vi "setUp.vi"(8 "error in (no error)":errorcluster, 11 "reference in":refnum<class "DFA Tester.lvclass">) -> (0 "error out":errorcluster, 3 "reference out":refnum<class "DFA Tester.lvclass">)   [LabVIEW 2017, in "DFA Tester.lvclass"]
doc: "setUp runs prior to the test method during test execution. Use this method to initialize any object data required by your tests."
uses:
  DFA Tester.lvclass
  C:/Program Files (x86)/National Instruments/LabVIEW 2017/vi.lib/addons/_JKI Toolkits/VI Tester/TestCase.llb/TestCase.lvclass
  Core/Assert API Components/Failure Actions.ctl
  DFA Tester.lvclass/DFA Tester.ctl
  <vilib>/addons/_JKI Toolkits/VI Tester/TestCase.llb/TestCase.lvclass
  Core/Assert API Components/Assert API Components.lvlib
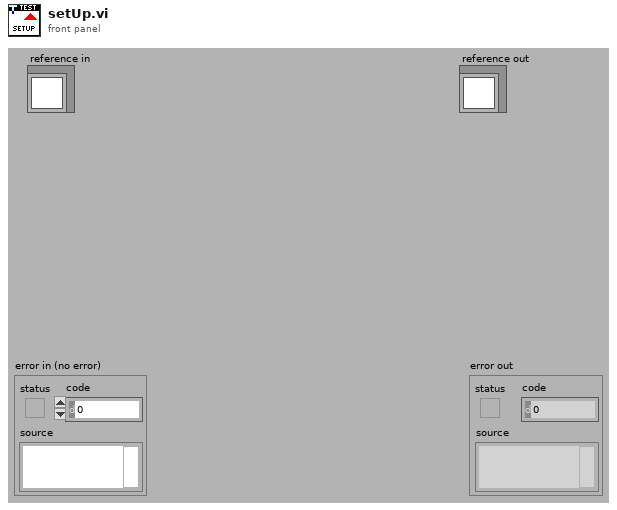
[diagram p1: front panel]
types:
  T1 = typedef "Assert API Components.lvlib/Failure Actions.ctl" = enum16{"None", "Log To File", "Pause Execution", "Abort Execution"}
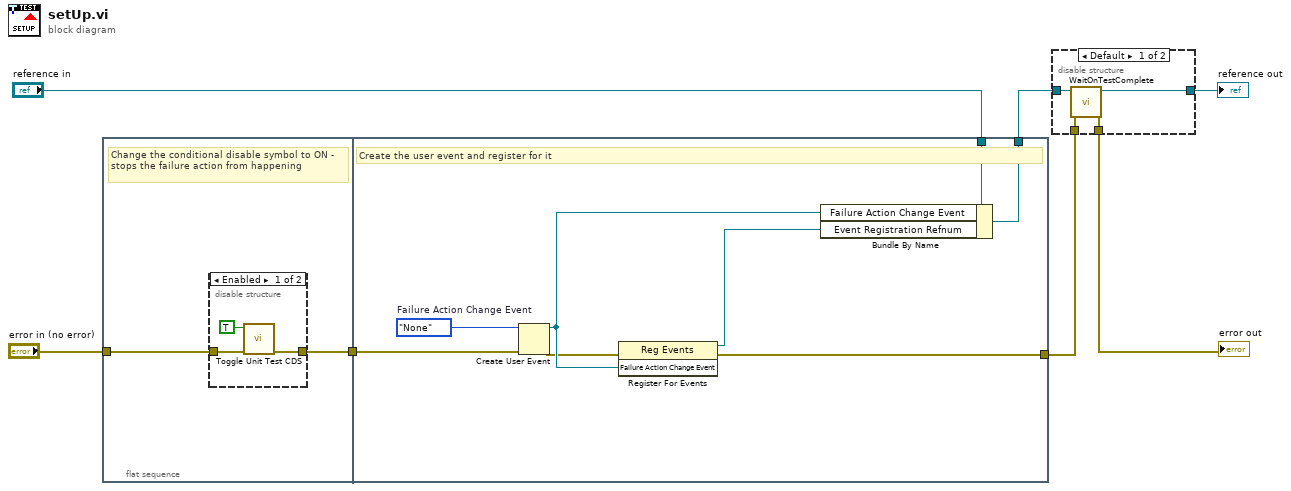
[diagram p0: block diagram]
diagram:
  n1 = flat-sequence {
    tunnel: "error in (no error)" -> [w9]
    tunnel: [w8] -> w1
    tunnel: "reference in" -> [w21]
    tunnel: [w20] -> w4
    tunnel: [w14] -> w2
    tunnel: w1 -> [w15]
    frame #0 {
      # "Change the conditional disable symbol to ON - stops the failure action from happening"
      n2 = disable-structure shown="Enabled" {
        disable-tunnel: w9 -> [w11 w13]
        disable-tunnel: [w10 w13] -> w8
        frame Enabled {
          n3 = call "Toggle Unit Test CDS.vi"("error in (no error)"=w11, "Requested State"=TRUE) -> ("error out"=w10:errorcluster)  [unwired: 9 in]
        }
        frame Disabled {
        }
      }
    }
    frame #1 {
      w19 = Failure_Actions."None"  # Failure Action Change Event
      # "Create the user event and register for it"
      n4 = Create User Event(user event datatype=w19, error in=w15) -> (user event=w18:refnum<user-event>, error out=w16:errorcluster)
      n5 = register-events(error in=w16, w18) -> (reference out=w17:refnum<event-registration>, error out=w14:errorcluster)  [unwired: 1 in]
      n6 = Bundle By Name(cluster=w21, "Failure Action Change Event"=w18, "Event Registration Refnum"=w17) -> (w20:refnum<class "DFA Tester.lvclass">)
    }
  }
  n7 = disable-structure shown="Default" {
    disable-tunnel: w2 -> [w25 w26]
    disable-tunnel: [w24 w26] -> w7
    disable-tunnel: [w23 w27] -> w5
    disable-tunnel: w4 -> [w22 w27]
    frame condition #0 (active) {
      n8 = call <vilib>:"WaitOnTestComplete.vi"("error in (no error)"=w25, "TestCase in"=w22) -> ("error out"=w24:errorcluster, "TestCase out"=w23:refnum<class "DFA Tester.lvclass">)  [unwired: 8 in]
    }
    frame condition #1 {
    }
  }
  "error out" <- w7
  "reference out" <- w5
